vi "@create.vi"(6 "autorun? (false)":bool, 7 "dotnet_system_exec in":refnum<class "dotnet_system_exec.lvclass">, 8 "error in (no error)":errorcluster, 9 "working directory (c:\\)":path=path "c:/", 10 "arguments (\"\")":string, 11 "command line (cmd.exe)":string="cmd.exe") -> (0 "error out":errorcluster, 2 "public events":T1, 3 "dotnet_system_exec out":refnum<class "dotnet_system_exec.lvclass">)   [LabVIEW 2020, in "JKI dotNET System Exec.lvlib" / "dotnet_system_exec.lvclass"]
doc: "Creates an instance of the .NET System Process. It configures the instance not to show a window but to redirect the stdout, stderr, and stdin so that LabVIEW can interface with them. Use the public events to register for the stdout and stderr events.\n\n-----------------------------------------------\nJKI .NET System Exec 1.0.0.6\nJavier Ruiz - JKI\nCopyright (c) 2021, JKI\njki.net"
uses:
  dotnet_system_exec.lvclass
  dotnet_system_exec.lvclass/dotnet_system_exec.ctl
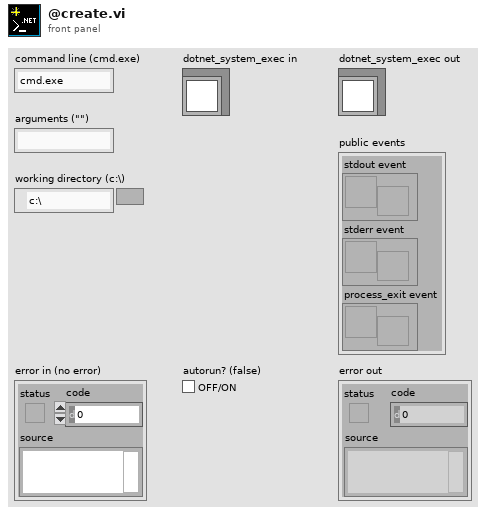
[diagram p1: front panel]
types:
  T1 = cluster{"stdout event":refnum<user-event>, "stderr event":refnum<user-event>, "process_exit event":refnum<user-event>}
  T2 = cluster{"StdOut Event":refnum<user-event>, "StdErr Event":refnum<user-event>, "ProcessExit Event":refnum<user-event>}
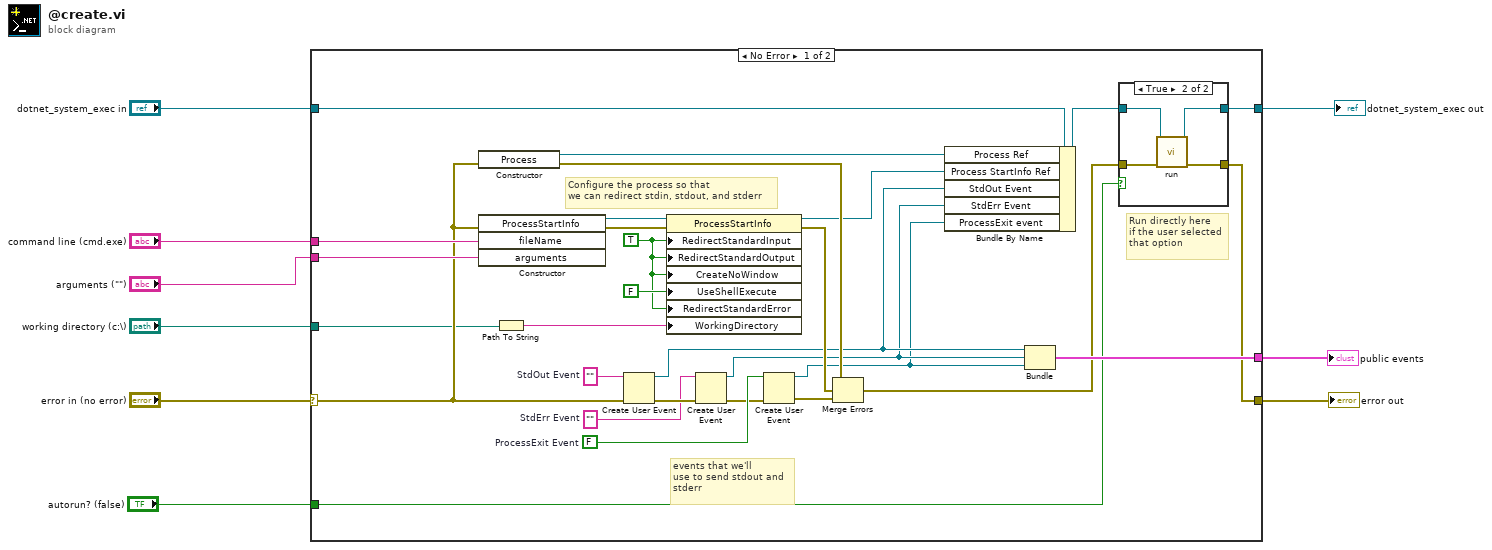
[diagram p0: block diagram]
diagram:
  n1 = case shown="No Error" "error in (no error)" {
    selector: "error in (no error)" -> [w23 w46]
    tunnel: [w15 w46] -> w8
    tunnel: [w17 w45] -> w6
    tunnel: "dotnet_system_exec in" -> [w29 w45]
    tunnel: "command line (cmd.exe)" -> [w32 _]
    tunnel: "arguments (\"\")" -> [w31 _]
    tunnel: "working directory (c:\\)" -> [w19 _]
    tunnel: [w22 _] -> w2
    tunnel: "autorun? (false)" -> [w14 _]
    frame No Error {
      w13 = FALSE  # ProcessExit Event
      w24 = ""  # StdErr Event
      w26 = ""  # StdOut Event
      w35 = TRUE ("RedirectStandardInput")
      # "Configure the process so that\nwe can redirect stdin, stdout, and stderr"
      # "events that we'll\nuse to send stdout and\nstderr"
      # "Run directly here\nif the user selected\nthat option"
      n2 = constructor class="Process"(error in=w23) -> (reference out=w28:refnum<k24>, error out=w34:errorcluster)  [unwired: 2 in, 1 out]
      n3 = constructor class="ProcessStartInfo"(error in=w23, "fileName"=w32, "arguments"=w31) -> (reference out=w37:refnum<k24>, error out=w38:errorcluster)  [unwired: 2 in, 3 out]
      n4 = Path To String(path=w19) -> (string=w30:string)
      n5 = Create User Event(user event datatype=w26, error in=w23) -> (user event=w21:refnum<user-event>, error out=w25:errorcluster)
      n6 = property class="ProcessStartInfo"(reference=w37, error in=w38, "RedirectStandardInput"=w35, "RedirectStandardOutput"=w35, "CreateNoWindow"=w35, "UseShellExecute"=FALSE, "RedirectStandardError"=w35, "WorkingDirectory"=w30) -> (reference out=w27:refnum<k24>, error out=w33:errorcluster)
      n7 = Create User Event(user event datatype=w24, error in=w25) -> (user event=w20:refnum<user-event>, error out=w12:errorcluster)
      n8 = Create User Event(user event datatype=w13, error in=w12) -> (user event=w10:refnum<user-event>, error out=w11:errorcluster)
      n9 = Merge Errors(w34, w33, w11) -> (w16:errorcluster)
      n10 = Bundle By Name(cluster=w29, "Process Ref"=w28, "Process StartInfo Ref"=w27, "StdOut Event"=w21, "StdErr Event"=w20, "ProcessExit event"=w10) -> (w18:refnum<class "dotnet_system_exec.lvclass">)
      n11 = Bundle("StdOut Event"=w21, "StdErr Event"=w20, "ProcessExit Event"=w10) -> (w22:T2)  [unwired: 1 in]
      n12 = case shown="True" w14 {
        tunnel: w18 -> [w40 w44]
        tunnel: [w40 w43] -> w17
        tunnel: w16 -> [w39 w42]
        tunnel: [w39 w41] -> w15
        frame False {
        }
        frame True {
          n13 = call "run.vi"("error in (no error)"=w42, "dotnet_system_exec in"=w44) -> ("error out"=w41:errorcluster, "dotnet_system_exec out"=w43:refnum<class "dotnet_system_exec.lvclass">)  [unwired: 8 in]
        }
      }
    }
    frame Error {
    }
  }
  "error out" <- w8
  "dotnet_system_exec out" <- w6
  "public events" <- w2
